vi "SPU_Set_Sampling_Parameter_for_Measure.vi"(0 "引用":refnum<k24>, 1 "startwave":dbl, 2 "stopwave":dbl, 3 "speed":dbl, 4 "triggerstep":dbl, 5 "错误输入（无错误）":errorcluster) -> (14 "引用输出":refnum<k24>, 19 "error IO":errorcluster)   [LabVIEW 2017]
uses:
  D:/test/FULLband-sts/Fullband_Sample/DLL/InstrumentDLL.dll
  DLL/InstrumentDLL.dll
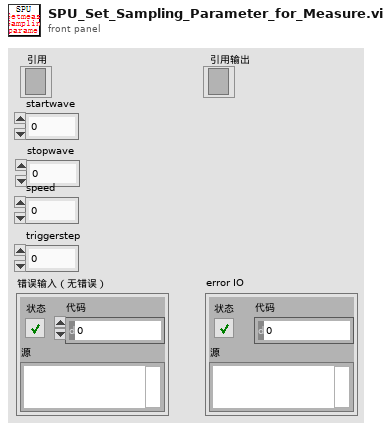
[diagram p1: front panel]
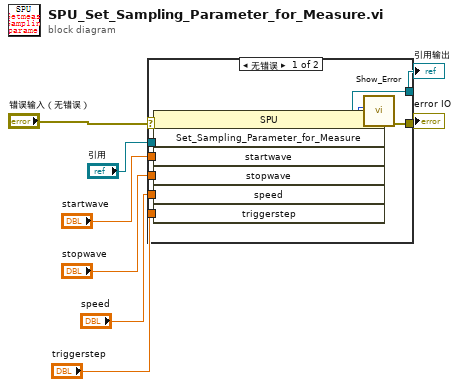
[diagram p0: block diagram]
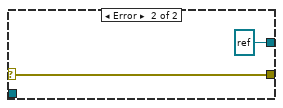
[diagram p2: hidden frame]
diagram:
  n1 = case shown="无错误" "错误输入（无错误）" {
    selector: "错误输入（无错误）" -> [_ w19]
    tunnel: [w15 w19] -> w6
    tunnel: [w14 refnum<k24> refnum ("new reference")] -> w7
    tunnel: "引用" -> [w13 _]
    tunnel: "startwave" -> [w12 _]
    tunnel: "stopwave" -> [w11 _]
    tunnel: "speed" -> [w10 _]
    tunnel: "triggerstep" -> [w9 _]
    frame No Error {
      n2 = invoke class="SPU" method="Set_Sampling_Parameter_for_Measure"(reference=w13, "startwave"=w12, "stopwave"=w11, "speed"=w10, "triggerstep"=w9) -> (reference out=w14:refnum<k24>, error out=w17:errorcluster, "Set_Sampling_Parameter_for_Measure"=w16:i32)  [unwired: 2 in, 4 out]
      n3 = call "Show_Error.vi"("error in (no error)"=w17, "Error"=w16) -> ("error out"=w15:errorcluster)  [unwired: 9 in]
    }
    frame Error {
    }
  }
  "引用输出" <- w7
  "error IO" <- w6
